vi "Flow Out P&F.vi"() -> ()   [LabVIEW 2017]
panel:
  out "Flow Out":dbl
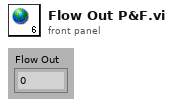
[diagram p1: front panel]
diagram:
